vi "Read.vi"(8 "error in (no error)":errorcluster, 10 "key":string, 11 "Object Dictionary in":refnum<class "objdict.lvclass">) -> (0 "error out":errorcluster, 1 "Object ref":refnum<data-value>, 3 "Object Dictionary out":refnum<class "objdict.lvclass">, 4 "found":bool)   [LabVIEW 2015, in "objdict.lvclass"]
doc: "Reads the Data Value Reference holding the object assigned to the specified key. Use this DVR with the In Place Element Structure to access or modify the object. If you want to remove the object from the dictionary instead of merely accessing it, use <b>Remove.vi</b>, instead.\n\nThis VI is part of a code pattern for accessing objects in the dictionary. Drop <b>Use Object in Dictionary.vit</b> from the palette."
uses:
  objdict.lvclass
  objdict.lvclass/objdict.ctl
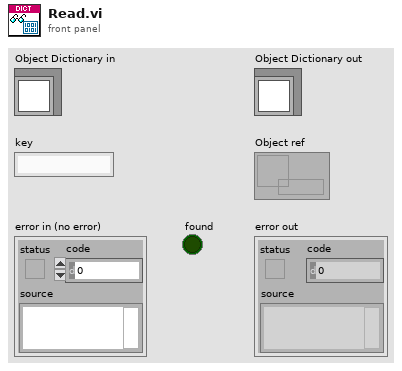
[diagram p1: front panel]
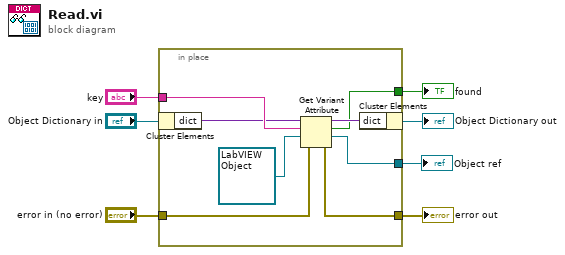
[diagram p0: block diagram]
diagram:
  n1 = in-place {
    in-place-border: [w14] -> w5
    in-place-border: "error in (no error)" -> [w15]
    in-place-border: "key" -> [w12]
    in-place-border: [w11] -> w2
    in-place-border: [w8] -> w1
    n2 = in-place-cluster #1("Object Dictionary in") -> ("dict"=w10:variant)
    n3 = Get Variant Attribute(Variant=w10, name=w12, default value (empty Variant)=refnum<data-value> refnum ("data value reference"), error in=w15) -> (duplicate Variant=w13:variant, found=w11:bool, value=w8:refnum<data-value>, error out=w14:errorcluster)
    n4 = in-place-cluster #1("dict"=w13) -> (→"Object Dictionary out":refnum<class "objdict.lvclass">)
  }
  "error out" <- w5
  "found" <- w2
  "Object ref" <- w1
